vi "Bind Method Query.vi"(11 "gRPCid server in":T1) -> (0 "error out":errorcluster, 2 "User Event out":refnum<user-event>, 3 "gRPCid server out":T1)   [LabVIEW 2019, in "OOP Server.lvclass"]
uses:
  OOP Server.lvclass
  gRPC interface/Server API/typeDefs/gRPCId Cluster.ctl
  gRPC interface/Server API/typeDefs/grpcId.ctl
  616620f9-6bbe-466a-af51-04bcc3596ea0.vi
  gRPC interface/gprc-lvsupport.lvlib
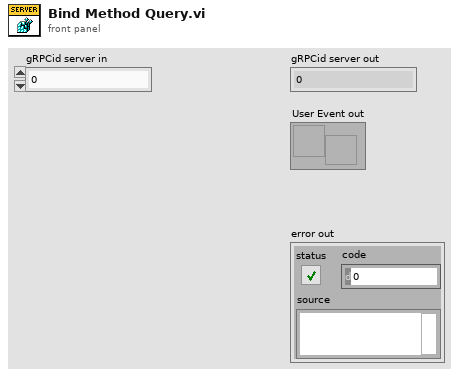
[diagram p1: front panel]
types:
  T1 = typedef "gprc-lvsupport.lvlib/grpcId.ctl" = u64
  T2 = typedef "gprc-lvsupport.lvlib/gRPCId Cluster.ctl" = cluster{"gRPCid":T1}
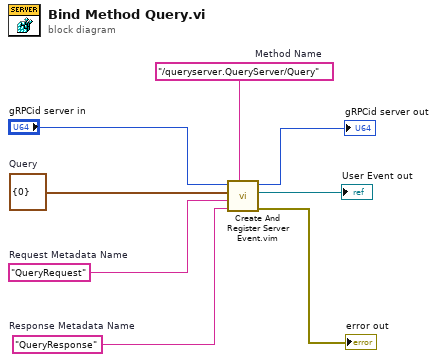
[diagram p0: block diagram]
diagram:
  w4 = "QueryResponse"  # Response Metadata Name
  w7 = T2 {"gRPCid"=0}  # Query
  w5 = "QueryRequest"  # Request Metadata Name
  w6 = "/queryserver.QueryServer/Query"  # Method Name
  n1 = call "Create And Register Server Event.vim"("Method name"=w6, "Response Metadata Name"=w4, "Request Metadata Name"=w5, "event in"=w7, "gRPCid server in"="gRPCid server in") -> ("error out"=→"error out":errorcluster, "event"=→"User Event out":refnum<user-event>, "gRPCid server out"=→"gRPCid server out":T1)  [unwired: 4 in]
